vi "Unescape JSON.vi"(11 "Escaped JSON":string) -> (3 "Unescaped JSON":string)   [LabVIEW 2015, in "NI_JSON Parsing.lvlib"]
uses:
  NI_JSON Parsing.lvlib
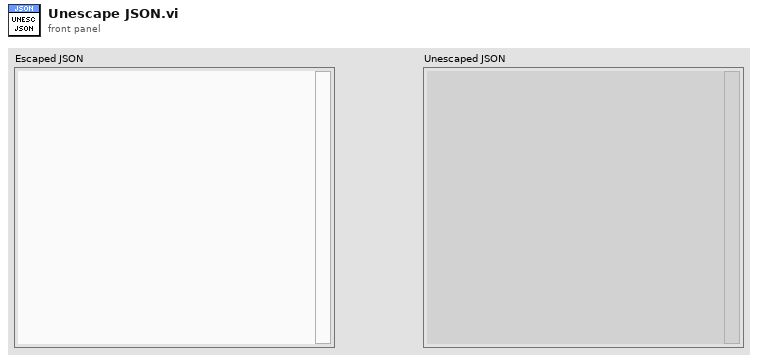
[diagram p1: front panel]
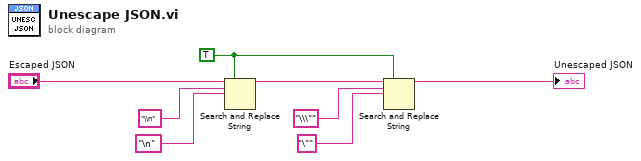
[diagram p0: block diagram]
diagram:
  w2 = TRUE ("replace all? (F)")
  n1 = Search and Replace String(replace all?=w2, input string="Escaped JSON", search string="\\n", replace string="\n") -> (result string=w3:string)  [unwired: 4 in, 3 out]
  n2 = Search and Replace String(replace all?=w2, input string=w3, search string="\\\"", replace string="\"") -> (result string=→"Unescaped JSON":string)  [unwired: 4 in, 3 out]
